vi "TextFit_Shrink next letter.vi"(7 "Font Size":T3, 8 "Error":errorcluster, 9 "Do Not Shrink":bool, 10 "Reset Prioity":bool, 11 "Character Array":T1[](array[typedef])) -> (0 "Error Out":errorcluster, 2 "All Items Shrunk Out":bool, 3 "Character Array Out":T1[](array[typedef]))   [LabVIEW 2014]
doc: "Compresses the next letter in the priority list"
uses:
  Controls/Cluster/Cluster_Character Size and Priority Data.ctl
  Controls/String_Picture/String Char Normal.ctl
  Controls/Enum/ENUM_Font Size Select.ctl
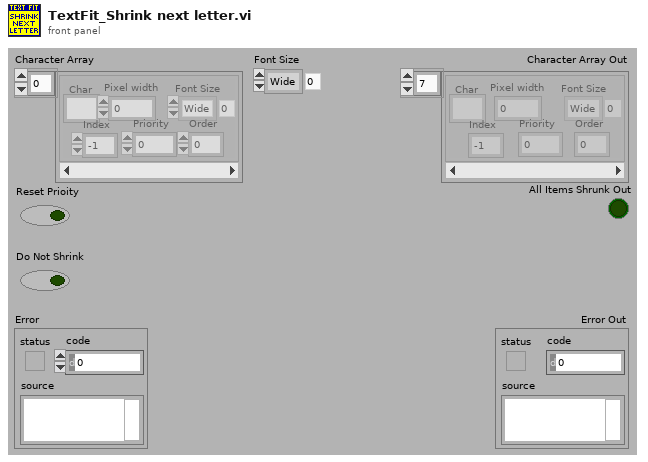
[diagram p1: front panel]
types:
  T1 = typedef "Cluster_Character Size and Priority Data.ctl" = cluster{"Char":T2, "Font Size":T3, "Pixel width":i32, "Priority":i32, "Order":i32, "Index":i32}
  T2 = typedef "String Char Normal.ctl" = string
  T3 = typedef "ENUM_Font Size Select.ctl" = enum16{"Wide", "Med", "Thin"}
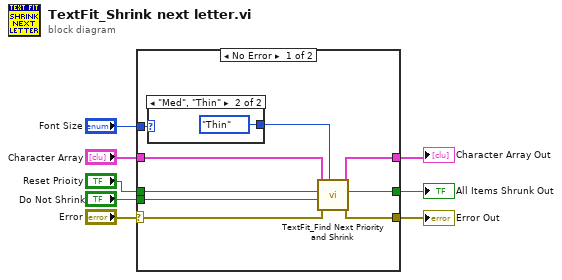
[diagram p0: block diagram]
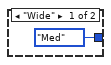
[diagram p2: hidden frame]
diagram:
  n1 = case shown="No Error" "Error" {
    selector: "Error" -> [w11 w20]
    tunnel: [w17 w20] -> w8
    tunnel: "Character Array" -> [w16 w21]
    tunnel: "Font Size" -> [w15 _]
    tunnel: [w13 w21] -> w5
    tunnel: [w12 _] -> w4
    tunnel: "Do Not Shrink" -> [w10 _]
    tunnel: "Reset Prioity" -> [w9 _]
    frame No Error {
      n2 = case shown="\"Med\", \"Thin\"" w15 {
        tunnel: [ENUM_Font_Size_Select."Med" ("Font Size Select") ENUM_Font_Size_Select."Thin" ("Font Size Select")] -> w14
        frame "Wide" {
        }
        frame "Med", "Thin" {
        }
      }
      n3 = call "TextFit_Find Next Priority and Shrink.vi"("Font Size"=w14, "Error"=w11, "Do Not Shrink"=w10, "Reset Prioity"=w9, "Array"=w16) -> ("Error Out"=w17:errorcluster, "All Items Shrunk Out"=w12:bool, "Array Out"=w13:T1[])  [unwired: 4 in]
    }
    frame Error {
    }
  }
  "Error Out" <- w8
  "All Items Shrunk Out" <- w4
  "Character Array Out" <- w5
